vi "Set Flip Vertical.vi"(8 "error in (no error)":errorcluster, 10 "Flip Vertical":bool, 11 "senseHatDisplay in":refnum<class "RPI.SenseHat.Display.lvclass">) -> (0 "error out":errorcluster, 3 "senseHatDisplay out":refnum<class "RPI.SenseHat.Display.lvclass">)   [LabVIEW 2020, in "RPI.SenseHat.Display.lvlib" / "RPI.SenseHat.Display.lvclass"]
doc: "Set to true to mirror the display vertically."
uses:
  RPI.SenseHat.Display.lvclass
  RPI.SenseHat.Display.lvclass/RPI.SenseHat.Display.ctl
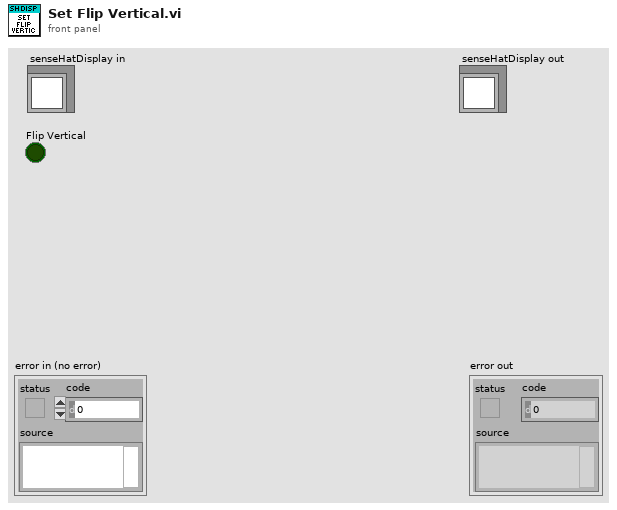
[diagram p1: front panel]
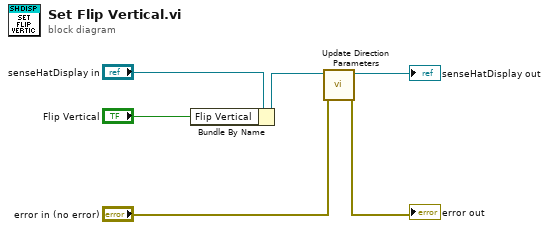
[diagram p0: block diagram]
diagram:
  n1 = Bundle By Name(cluster="senseHatDisplay in", "Flip Vertical"="Flip Vertical") -> (w4:refnum<class "RPI.SenseHat.Display.lvclass">)
  n2 = call "Update Direction Parameters.vi"("error in (no error)"="error in (no error)", "senseHatDisplay in"=w4) -> ("error out"=→"error out":errorcluster, "senseHatDisplay out"=→"senseHatDisplay out":refnum<class "RPI.SenseHat.Display.lvclass">)  [unwired: 8 in]
